vi "HTTP-OPTIONS.vi"(8 "error in (no error)":errorcluster, 10 "req":string, 11 "URL":string="http://localhost:24414") -> (0 "error out":errorcluster, 2 "body":string, 3 "header":string)   [LabVIEW 2020]
uses:
  <vilib>/regexp/Match Regular Expression.xnode
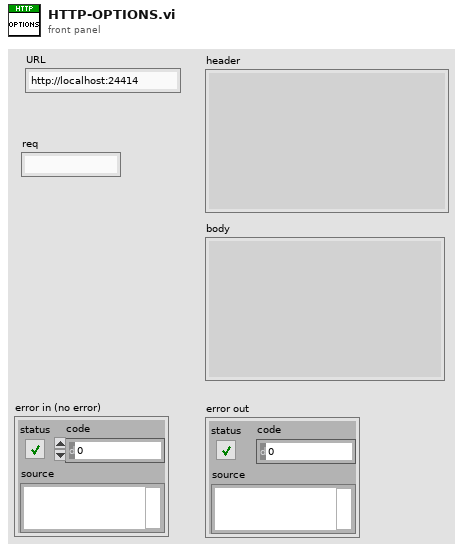
[diagram p1: front panel]
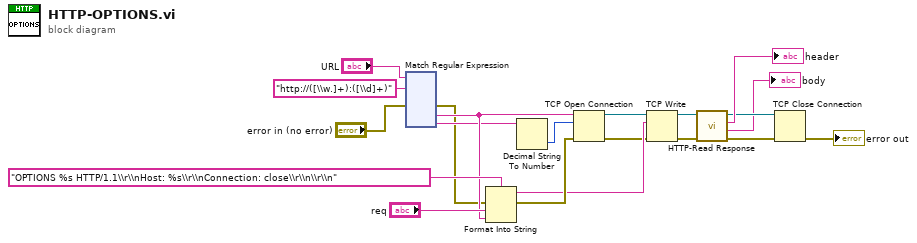
[diagram p0: block diagram]
diagram:
  n1 = xnode "Match Regular Expression"("input string"="URL", "regular expression"="http://([\\w.]+):([\\d]+)", "error in"="error in (no error)") -> ("error out"=w8:errorcluster, "submatch 1"=w11:string, "submatch 2"=w10:string)  [unwired: 3 in, 4 out]
  n2 = Format Into String(format string="OPTIONS %s HTTP/1.1\\r\\nHost: %s\\r\\nConnection: close\\r\\n\\r\\n" ("data in"), error in=w8, "req", w11) -> (resulting string=w17:string, error out=w18:errorcluster)  [unwired: 1 in]
  n3 = Decimal String To Number(string=w10) -> (number=w9:i32)  [unwired: 2 in, 1 out]
  n4 = TCP Open Connection(address=w11, remote port or service name=w9, error in (no error)=w18) -> (connection ID=w7:refnum<k5>, error out=w6:errorcluster)  [unwired: 2 in]
  n5 = TCP Write(connection ID=w7, data in=w17, error in (no error)=w6) -> (connection ID out=w4:refnum<k5>, error out=w5:errorcluster)  [unwired: 1 in, 1 out]
  n6 = call "HTTP-Read Response.vi"("error in (no error)"=w5, "TCP Network Connection in"=w4) -> ("error out"=w2:errorcluster, "Body"=→"body":string, "Header"=→"header":string, "TCP Network Connection out"=w3:refnum<k5>)  [unwired: 6 in]
  n7 = TCP Close Connection(connection ID=w3, error in (no error)=w2) -> (error out=→"error out":errorcluster)  [unwired: 1 in, 1 out]
